vi "Read Conversion Time.vi"(8 "error in":errorcluster, 11 "NI 9212 in":refnum<class "NI 9212.lvclass">) -> (0 "error out":errorcluster, 2 "conversion time":T1, 3 "NI 9212 out":refnum<class "NI 9212.lvclass">)   [LabVIEW 2017, in "Scan Engine Scripting.lvlib" / "NI 9212.lvclass"]
doc: "Reads the conversion time from the module."
uses:
  NI 9212.lvclass
  NI 9212 Conversion Time.ctl
  NI 9212.lvclass/NI 9212.ctl
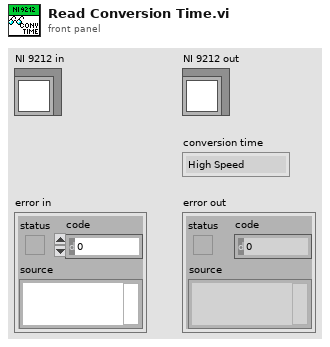
[diagram p1: front panel]
types:
  T1 = typedef "Scan Engine Scripting.lvlib/NI 9212.lvclass/NI 9212 Conversion Time.ctl" = enum16{"High Speed", "Best 60 Hz Rejection", "Best 50 Hz Rejection", "High Resolution"}
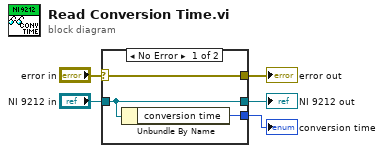
[diagram p0: block diagram]
diagram:
  n1 = case shown="No Error" "error in" {
    selector: "error in" -> [w8 w9]
    tunnel: [w8 w9] -> w4
    tunnel: [w7 w10] -> w2
    tunnel: "NI 9212 in" -> [w7 w10]
    tunnel: [w6 _] -> w1
    frame No Error {
      n2 = Unbundle By Name(w7) -> ("conversion time"=w6:T1)
    }
    frame Error {
    }
  }
  "error out" <- w4
  "NI 9212 out" <- w2
  "conversion time" <- w1
